vi "Open Connection to All - Type Code Array.vi"(8 "Error In":errorcluster, 10 "Type code Array":i32[](array[numeric]), 11 "URL array":string[](array[string])) -> (0 "Error Out":errorcluster, 1 "Error Status":bool, 2 "Type code Array":i32[](array[numeric]), 3 "Array of SV Refnums":refnum<k21>[](array[refnum]))   [LabVIEW 2014]
doc: "<B>Copyright</B>: (c) MHWirth 2015. All rights reserved.\n\nThis VI opens connection to all shared variables that are specified using URL and Type arrays.\n\nIf the type is unknown (Error 7001) or read variable function is errorenous, the loop stops and Error Status is True. \n\n<B>Defined Types</B>:\nCode 1. Boolean\nCode 2 to 5. Int8/16/32/64\nCode 6 to 9. UInt8/16/32/64\nCode 10. Double\nCode 11. Single-precision\nCode 12. String\nCode 13 to 24. 1D array of xxx\nCode 25 to 36. 2D array of xxxs\n\n<B>Error 7001</B>: Unknown Data Type - Type Code Array (Int32) contains -1 indicating an unknown data type."
panel:
  out "Status":string
  out "Number of Deployed SV":i32
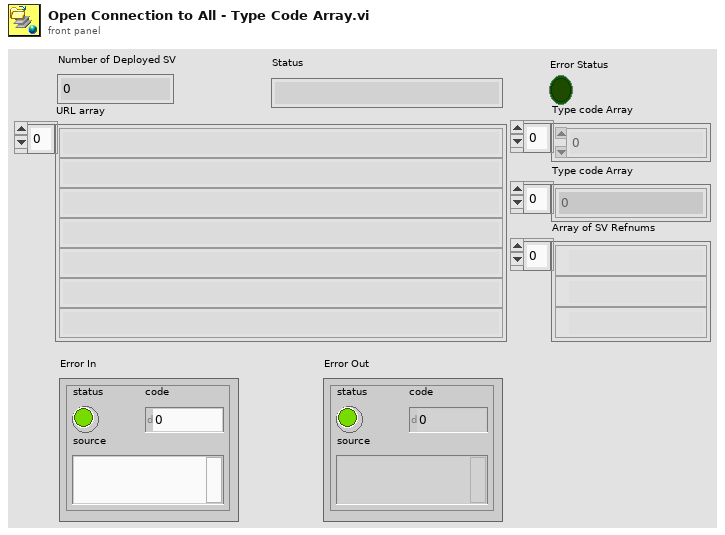
[diagram p1: front panel]
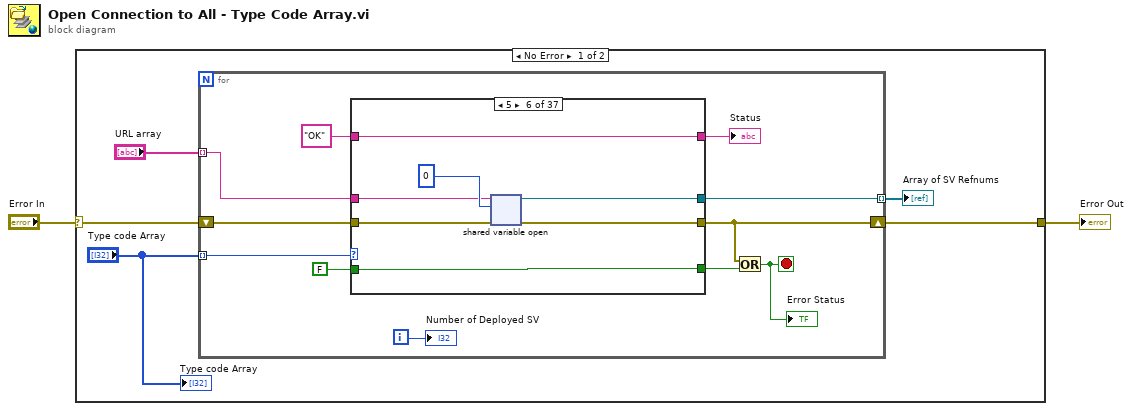
[diagram p0: block diagram]
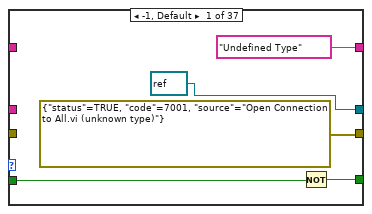
[diagram p2: hidden frame]
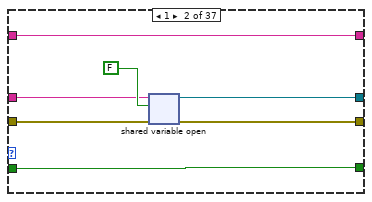
[diagram p3: hidden frame]
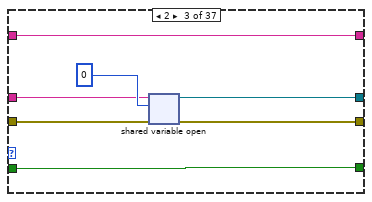
[diagram p4: hidden frame]
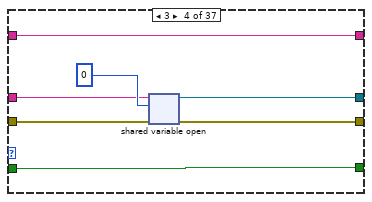
[diagram p5: hidden frame]
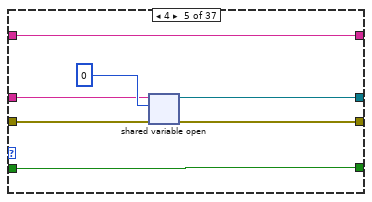
[diagram p6: hidden frame]
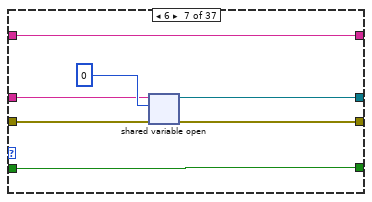
[diagram p7: hidden frame]
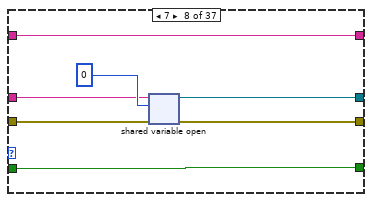
[diagram p8: hidden frame]
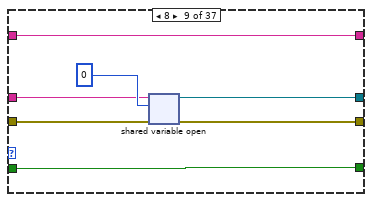
[diagram p9: hidden frame]
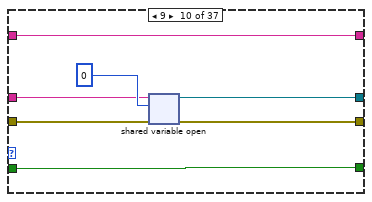
[diagram p10: hidden frame]
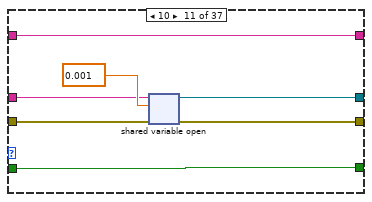
[diagram p11: hidden frame]
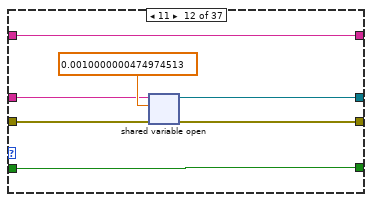
[diagram p12: hidden frame]
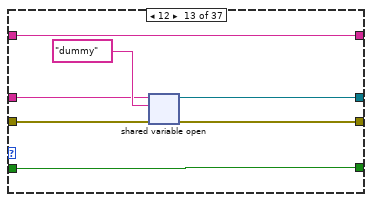
[diagram p13: hidden frame]
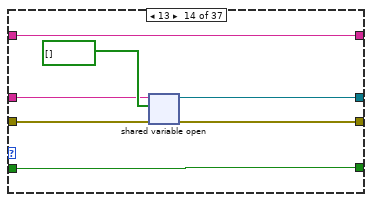
[diagram p14: hidden frame]
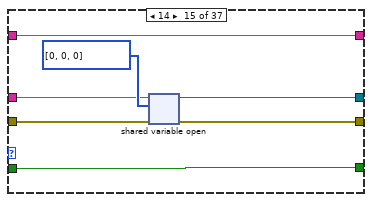
[diagram p15: hidden frame]
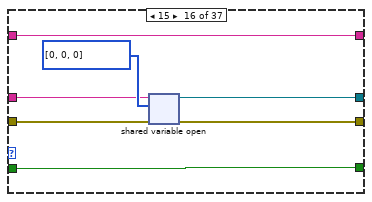
[diagram p16: hidden frame]
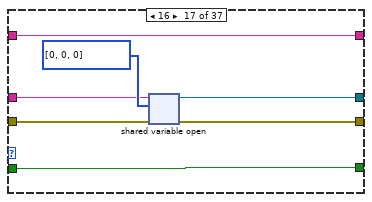
[diagram p17: hidden frame]
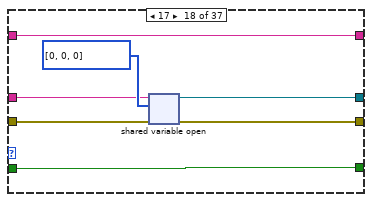
[diagram p18: hidden frame]
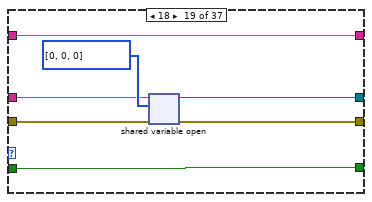
[diagram p19: hidden frame]
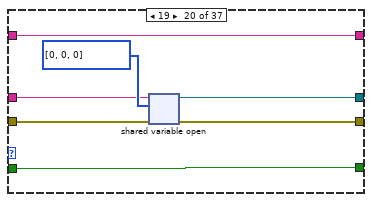
[diagram p20: hidden frame]
diagram:
  n1 = case shown="No Error" "Error In" {
    selector: "Error In" -> [w7 w276]
    tunnel: [w6 w276] -> w1
    frame No Error {
      n2 = for {
        shift-right: [w9] -> w6
        shift-left: w7 -> [w18]
        tunnel: "Type code Array" -> [w13] mode=indexing
        tunnel: "URL array" -> [w12] mode=indexing
        tunnel: [w11] -> w4 mode=indexing
        i -> [w17]
        stop <- w8 stop-if-true
        n3 = case shown="5" w13 {
          tunnel: w18 -> [_ w29 w36 w43 w50 w57 w64 w71 w78 w85 w92 w99 w107 w113 w120 w127 w134 w141 w148 w155 w162 w169 w176 w183 w190 w197 w204 w211 w218 w225 w232 w239 w246 w253 w260 w267 w274]
          tunnel: [errorcluster {"status"=TRUE, "code"=7001, "source"="Open Connection to All.vi (unknown type)"} ("error constant") w26 w33 w40 w47 w54 w61 w68 w75 w82 w89 w96 w103 w110 w117 w124 w131 w138 w145 w152 w159 w166 w172 w180 w187 w194 w201 w208 w215 w222 w229 w236 w243 w250 w257 w264 w271] -> w9
          tunnel: ["Undefined Type" w28 w35 w42 w49 w56 w63 w70 w77 w84 w91 w98 w106 w112 w119 w126 w133 w140 w147 w154 w161 w168 w175 w182 w189 w196 w203 w210 w217 w224 w231 w238 w245 w252 w259 w266 w273] -> w16
          tunnel: "OK" -> [_ w28 w35 w42 w49 w56 w63 w70 w77 w84 w91 w98 w106 w112 w119 w126 w133 w140 w147 w154 w161 w168 w175 w182 w189 w196 w203 w210 w217 w224 w231 w238 w245 w252 w259 w266 w273]
          tunnel: FALSE -> [w22 w27 w34 w41 w48 w55 w62 w69 w76 w83 w90 w97 w105 w111 w118 w125 w132 w139 w146 w153 w160 w167 w174 w181 w188 w195 w202 w209 w216 w223 w230 w237 w244 w251 w258 w265 w272]
          tunnel: [w21 w27 w34 w41 w48 w55 w62 w69 w76 w83 w90 w97 w105 w111 w118 w125 w132 w139 w146 w153 w160 w167 w174 w181 w188 w195 w202 w209 w216 w223 w230 w237 w244 w251 w258 w265 w272] -> w10
          tunnel: w12 -> [_ w25 w32 w39 w46 w53 w60 w67 w74 w81 w88 w95 w102 w109 w116 w123 w130 w137 w144 w151 w158 w165 w173 w179 w186 w193 w200 w207 w214 w221 w228 w235 w242 w249 w256 w263 w270]
          tunnel: [refnum<k21> refnum w24 w31 w38 w45 w52 w59 w66 w73 w80 w87 w94 w101 w108 w115 w122 w129 w136 w143 w150 w157 w164 w171 w178 w185 w192 w199 w206 w213 w220 w227 w234 w241 w248 w255 w262 w269] -> w11
          frame -1, Default {
            n4 = Not(x=w22) -> (.not. x?=w21:bool)
          }
          frame 1 {
            n5 = shared-variable-open(w25, w29, FALSE) -> (w24:refnum<k21>, w26:errorcluster)  [unwired: 1 in]
          }
          frame 2 {
            n6 = shared-variable-open(w32, w36, i8 0) -> (w31:refnum<k21>, w33:errorcluster)  [unwired: 1 in]
          }
          frame 3 {
            n7 = shared-variable-open(w39, w43, i16 0) -> (w38:refnum<k21>, w40:errorcluster)  [unwired: 1 in]
          }
          frame 4 {
            n8 = shared-variable-open(w46, w50, 0) -> (w45:refnum<k21>, w47:errorcluster)  [unwired: 1 in]
          }
          frame 5 {
            n9 = shared-variable-open(w53, w57, i64 0) -> (w52:refnum<k21>, w54:errorcluster)  [unwired: 1 in]
          }
          frame 6 {
            n10 = shared-variable-open(w60, w64, u8 0) -> (w59:refnum<k21>, w61:errorcluster)  [unwired: 1 in]
          }
          frame 7 {
            n11 = shared-variable-open(w67, w71, u16 0) -> (w66:refnum<k21>, w68:errorcluster)  [unwired: 1 in]
          }
          frame 8 {
            n12 = shared-variable-open(w74, w78, u32 0) -> (w73:refnum<k21>, w75:errorcluster)  [unwired: 1 in]
          }
          frame 9 {
            n13 = shared-variable-open(w81, w85, u64 0) -> (w80:refnum<k21>, w82:errorcluster)  [unwired: 1 in]
          }
          frame 10 {
            n14 = shared-variable-open(w88, w92, 0.001) -> (w87:refnum<k21>, w89:errorcluster)  [unwired: 1 in]
          }
          frame 11 {
            n15 = shared-variable-open(w95, w99, sgl 0.001) -> (w94:refnum<k21>, w96:errorcluster)  [unwired: 1 in]
          }
          frame 12 {
            n16 = shared-variable-open(w102, w107, "dummy") -> (w101:refnum<k21>, w103:errorcluster)  [unwired: 1 in]
          }
          frame 13 {
            n17 = shared-variable-open(w109, w113, bool[] []) -> (w108:refnum<k21>, w110:errorcluster)  [unwired: 1 in]
          }
          frame 14 {
            n18 = shared-variable-open(w116, w120, i8[] [0, 0, 0]) -> (w115:refnum<k21>, w117:errorcluster)  [unwired: 1 in]
          }
          frame 15 {
            n19 = shared-variable-open(w123, w127, i16[] [0, 0, 0]) -> (w122:refnum<k21>, w124:errorcluster)  [unwired: 1 in]
          }
          frame 16 {
            n20 = shared-variable-open(w130, w134, i32[] [0, 0, 0]) -> (w129:refnum<k21>, w131:errorcluster)  [unwired: 1 in]
          }
          frame 17 {
            n21 = shared-variable-open(w137, w141, i64[] [0, 0, 0]) -> (w136:refnum<k21>, w138:errorcluster)  [unwired: 1 in]
          }
          frame 18 {
            n22 = shared-variable-open(w144, w148, u8[] [0, 0, 0]) -> (w143:refnum<k21>, w145:errorcluster)  [unwired: 1 in]
          }
          frame 19 {
            n23 = shared-variable-open(w151, w155, u16[] [0, 0, 0]) -> (w150:refnum<k21>, w152:errorcluster)  [unwired: 1 in]
          }
          frame 20 {
            n24 = shared-variable-open(w158, w162, u32[] [0, 0, 0]) -> (w157:refnum<k21>, w159:errorcluster)  [unwired: 1 in]
          }
          frame 21 {
            n25 = shared-variable-open(w165, w169, u64[] [0, 0, 0]) -> (w164:refnum<k21>, w166:errorcluster)  [unwired: 1 in]
          }
          frame 22 {
            n26 = shared-variable-open(w173, w176, dbl[] [0.0, 0.0, 0.0]) -> (w171:refnum<k21>, w172:errorcluster)  [unwired: 1 in]
          }
          frame 23 {
            n27 = shared-variable-open(w179, w183, sgl[] [0.0, 0.0, 0.0]) -> (w178:refnum<k21>, w180:errorcluster)  [unwired: 1 in]
          }
          frame 24 {
            n28 = shared-variable-open(w186, w190, string[] []) -> (w185:refnum<k21>, w187:errorcluster)  [unwired: 1 in]
          }
          frame 25 {
            n29 = shared-variable-open(w193, w197, bool[][] []) -> (w192:refnum<k21>, w194:errorcluster)  [unwired: 1 in]
          }
          frame 26 {
            n30 = shared-variable-open(w200, w204, i8[][] [[0, 0, 0]]) -> (w199:refnum<k21>, w201:errorcluster)  [unwired: 1 in]
          }
          frame 27 {
            n31 = shared-variable-open(w207, w211, i16[][] [[0, 0, 0]]) -> (w206:refnum<k21>, w208:errorcluster)  [unwired: 1 in]
          }
          frame 28 {
            n32 = shared-variable-open(w214, w218, i32[][] [[0, 0, 0]]) -> (w213:refnum<k21>, w215:errorcluster)  [unwired: 1 in]
          }
          frame 29 {
            n33 = shared-variable-open(w221, w225, i64[][] [[0, 0, 0]]) -> (w220:refnum<k21>, w222:errorcluster)  [unwired: 1 in]
          }
          frame 30 {
            n34 = shared-variable-open(w228, w232, u8[][] [[0, 0, 0]]) -> (w227:refnum<k21>, w229:errorcluster)  [unwired: 1 in]
          }
          frame 31 {
            n35 = shared-variable-open(w235, w239, u16[][] [[0, 0, 0]]) -> (w234:refnum<k21>, w236:errorcluster)  [unwired: 1 in]
          }
          frame 32 {
            n36 = shared-variable-open(w242, w246, u32[][] [[0, 0, 0]]) -> (w241:refnum<k21>, w243:errorcluster)  [unwired: 1 in]
          }
          frame 33 {
            n37 = shared-variable-open(w249, w253, u64[][] [[0, 0, 0]]) -> (w248:refnum<k21>, w250:errorcluster)  [unwired: 1 in]
          }
          frame 34 {
            n38 = shared-variable-open(w256, w260, dbl[][] [[0.0, 0.0, 0.0]]) -> (w255:refnum<k21>, w257:errorcluster)  [unwired: 1 in]
          }
          frame 35 {
            n39 = shared-variable-open(w263, w267, sgl[][] [[0.0, 0.0, 0.0]]) -> (w262:refnum<k21>, w264:errorcluster)  [unwired: 1 in]
          }
          frame 36 {
            n40 = shared-variable-open(w270, w274, string[][] []) -> (w269:refnum<k21>, w271:errorcluster)  [unwired: 1 in]
          }
        }
        "Status" <- w16
        n41 = Or(x=w9, y=w10) -> (x .or. y?=w8:bool)
        "Error Status" <- w8
        "Number of Deployed SV" <- w17
      }
      "Array of SV Refnums" <- w4
      "Type code Array" <- "Type code Array"
    }
    frame Error {
    }
  }
  "Error Out" <- w1
